vi "Test Maxscend SP4T.vi"() -> ()   [LabVIEW 2020, in "Maxscend SP4T.lvclass"]
uses:
  Maxscend SP4T.lvclass
  Controls/Change setting mode enum.ctl
  PIC-device/PIC-Device.lvclass
panel:
  out "Changes":cluster{"Name":string, "Value":string}[][](array[cluster])
  in  "y":bool
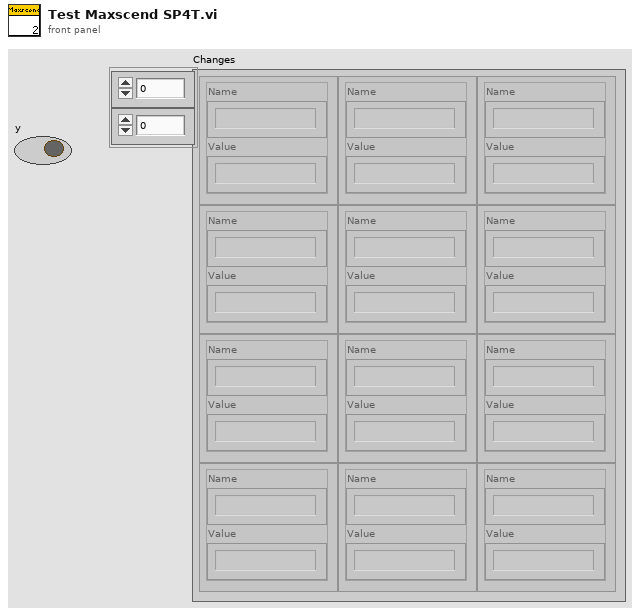
[diagram p1: front panel]
types:
  T1 = typedef "PIC-Device.lvclass/Change setting mode enum.ctl" = enum16{"Init", "Next", "Reset"}
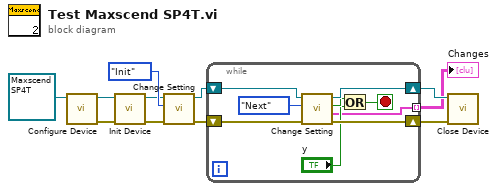
[diagram p0: block diagram]
diagram:
  n1 = call-dynamic "Configure Device.vi"("Maxscend SP4T in"=refnum<class "Maxscend SP4T.lvclass"> refnum ("Maxscend SP4T.lvclass")) -> ("error out"=w5:errorcluster, "Maxscend SP4T out"=w4:refnum<class "Maxscend SP4T.lvclass">)  [unwired: 9 in]
  n2 = call-dynamic "Init Device.vi"("error in (no error)"=w5, "NI DAQmx in"=w4) -> ("error out"=w3:errorcluster, "NI DAQmx out"=w2:refnum<class "Maxscend SP4T.lvclass">)  [unwired: 8 in]
  n3 = call-dynamic "Change Setting.vi"("error in (no error)"=w3, "Change setting mode"=Change_setting_mode_enum."Init", "NI DAQmx in"=w2) -> ("error out"=w10:errorcluster, "NI DAQmx out"=w11:refnum<class "Maxscend SP4T.lvclass">)  [unwired: 5 in, 2 out]
  n4 = while {
    shift-right: [w18] -> w9
    shift-left: w11 -> [w20]
    shift-right: [w17] -> w8
    shift-left: w10 -> [w19]
    tunnel: [w12] -> w6 mode=indexing
    stop <- w13 stop-if-true
    n5 = call-dynamic "Change Setting.vi"("error in (no error)"=w19, "Change setting mode"=Change_setting_mode_enum."Next", "NI DAQmx in"=w20) -> ("error out"=w17:errorcluster, "Changes"=w12:cluster{"Name":string, "Value":string}[], "Last setting"=w15:bool, "NI DAQmx out"=w18:refnum<class "Maxscend SP4T.lvclass">)  [unwired: 5 in]
    n6 = Or(x=w15, y="y") -> (x .or. y?=w13:bool)
  }
  "Changes" <- w6
  n7 = call-dynamic "Close Device.vi"("error in (no error)"=w8, "NI DAQmx in"=w9) -> ()  [unwired: 8 in, 2 out]
